vi "Initialize Device.vi"(8 "error in (no error)":errorcluster, 9 "Number of Axes":i32, 10 "VISA resource name":refnum<visa-resource-name>, 11 "Simulated in":refnum<class "Simulated-TS.lvclass">) -> (0 "error out":errorcluster, 3 "Simulated out":refnum<class "Simulated-TS.lvclass">)   [LabVIEW 2019, in "Simulated-TS.lvclass"]
uses:
  Simulated-TS.lvclass
  Simulated-TS.lvclass/Simulated-TS.ctl
  <vilib>/numeric/Random Number (Range) DBL.vi
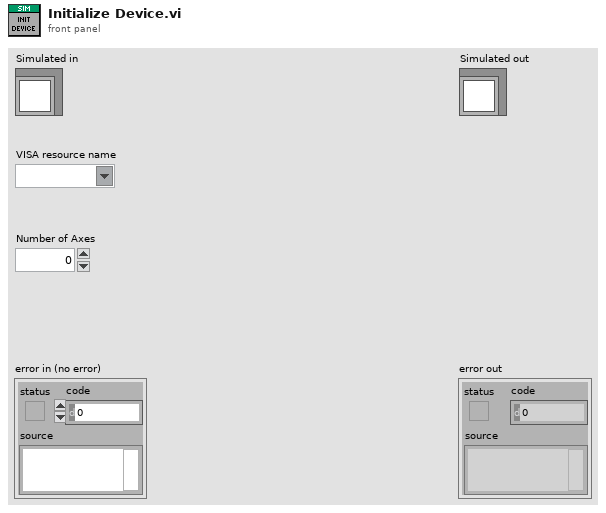
[diagram p1: front panel]
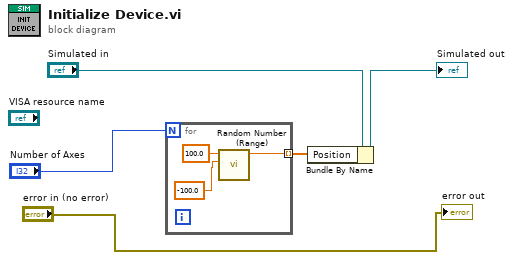
[diagram p0: block diagram]
diagram:
  n1 = for {
    N: "Number of Axes" -> [_]
    tunnel: [w6] -> w2 mode=indexing
    n2 = call-poly <vilib>:"Random Number (Range).vi"("lower bound (0)"=-100.0, "upper bound (100)"=100.0) -> ("number"=w6:dbl)  [unwired: 9 in]
  }
  n3 = Bundle By Name(cluster="Simulated in", "Position"=w2) -> (→"Simulated out":refnum<class "Simulated-TS.lvclass">)
  "error out" <- "error in (no error)"
